vi "Create.vi"(4 "DataProc Options":T1, 6 "Parent Name":string, 8 "error in (no error)":errorcluster, 10 "Group":refnum<class "Group DBL.lvclass">) -> (0 "error out":errorcluster, 3 "Data Processor Module out":refnum<class "Data Processor Module.lvclass">)   [LabVIEW 2020, in "VolatusData.lvlib" / "Data Processor Module.lvclass"]
uses:
  Data Processor Module.lvclass
  lv-vecto/Vecto/Group DBL/Group DBL.lvclass
  C:/dev/lv20CE/relink/lv-vecto/Vecto/Group/Group.lvclass
  DataProc Options.ctl
  lv-vecto/Vecto/Group/Group.lvclass/Group.ctl
  lv-vecto/Vecto/Group Config/Group Config.lvclass/Group Config.ctl
  Data Processor Module.lvclass/Data Processor Module.ctl
  lv-vecto/Vecto/Group/Group.lvclass
  VolatusData.lvlib
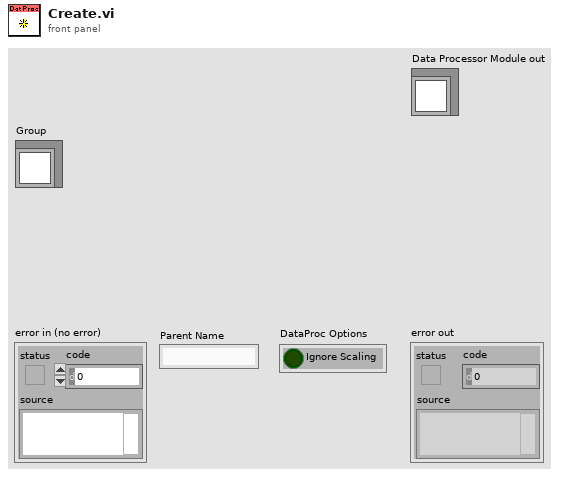
[diagram p1: front panel]
types:
  T1 = typedef "VolatusData.lvlib/DataProc Options.ctl" = cluster{"Ignore Scaling":bool}
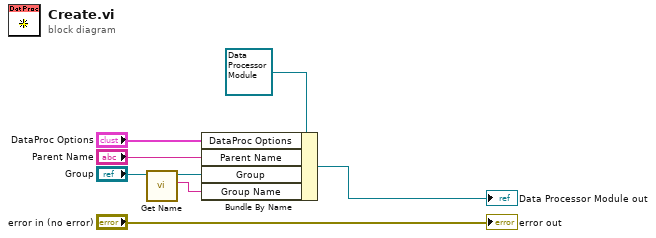
[diagram p0: block diagram]
diagram:
  n1 = call "Get Name.vi"("GroupAbstract in"="Group") -> ("Name"=w1:string, "GroupAbstract out"=w2:refnum<class "Group DBL.lvclass">)  [unwired: 8 in, 1 out]
  n2 = Bundle By Name(cluster=refnum<class "Data Processor Module.lvclass"> refnum ("Data Processor Module in"), "DataProc Options"="DataProc Options", "Parent Name"="Parent Name", "Group"=w2, "Group Name"=w1) -> (→"Data Processor Module out":refnum<class "Data Processor Module.lvclass">)
  "error out" <- "error in (no error)"
